vi "LAS.vi"() -> ()   [LabVIEW 2014, in "Panels.lvlib"]
uses:
  Panels.lvlib
  CSlibraries-extern/DimLVEvent/DimIndicators/DimIndicators.lvlib
  CSCore/CSSystem/CoreLib/CoreLib.lvlib
  CSlibraries/UtilityLib/UtilityLib.valueStatus.ctl
  CSlibraries/UtilityLib/UtilityLib.lvlib
  CSlibraries-extern/DimLVEvent/LVDimInterface/LVDimInterface.lvlib
  Instance           1 11Saved   LAS .vi
  CSlibraries-extern/DimLVEvent/DimIndicators/DimIndicators.numericType.ctl
  CSlibraries-extern/DimLVEvent/DimIndicators/DimIndicators.numericArrayType.ctl
  CSlibraries-extern/DimLVEvent/DimIndicators/DimIndicators.anyType.ctl
panel:
  in  "LASOuterQ-_SetValueInfoData":T1={"data"=[], "no link"=TRUE, "quality"=-1, "timeStamp"=0.0}
  in  "LASOuterQ+_SetValueInfoData":T1={"data"=[], "no link"=TRUE, "quality"=-1, "timeStamp"=0.0}
  in  "LASInnerQ-_SetValueInfoData":T1={"data"=[], "no link"=TRUE, "quality"=-1, "timeStamp"=0.0}
  in  "LASOuterQ-_SetData":T1={"data"=[], "no link"=TRUE, "quality"=-1, "timeStamp"=0.0}
  in  "LASOuterQ+_SetData":T1={"data"=[], "no link"=TRUE, "quality"=-1, "timeStamp"=0.0}
  in  "LASInnerQ-_SetData":T1={"data"=[], "no link"=TRUE, "quality"=-1, "timeStamp"=0.0}
  in  "LASOuterQ-_MonData":T2={"data"=inf, "no link"=TRUE, "quality"=-1, "timeStamp"=0.0}
  in  "LASOuterQ+_MonData":T2={"data"=inf, "no link"=TRUE, "quality"=-1, "timeStamp"=0.0}
  in  "LASInnerQ-_MonData":T2={"data"=inf, "no link"=TRUE, "quality"=-1, "timeStamp"=0.0}
  in  "LASOuterQ-":bool
  in  "LASOuterQ+":bool
  out "LASOuterQ+_Mon":dbl=inf format="%.4f"
  out "LASOuterQ-_Mon":dbl=inf format="%.4f"
  in  "LASInnerQ+":bool
  in  "LASAccel2":bool
  out "LASAccel2_Mon":dbl=inf format="%.4f"
  in  "LASInnerQ-":bool
  out "LASInnerQ-_Mon":dbl=inf format="%.4f"
  in  "SetFileLocation_Data":T3={"data"="NOLINK", "no link"=TRUE, "quality"=-1, "timeStamp"=0.0}
  in  "SetFileLocation":path=path "\\\\intranet\\Files/projects/lebit/Data Exchange/data/PenningEjectControl"
  in  "LASAccel3":bool
  in  "LASAccel4":bool
  in  "LASAccel1":bool
  out "LASAccel4_Mon":dbl=inf format="%.4f"
  out "LASAccel3_Mon":dbl=inf format="%.4f"
  out "i ref out":refnum<vi>
  in  "Last Loaded File_Data":T3={"data"="NOLINK", "no link"=TRUE, "quality"=-1, "timeStamp"=0.0}
  out "FileUpToDate":bool=TRUE caption="Parameter Changed"
  in  "Close All Panels":bool
  in  "LASAccel2_SetValueInfoData":T1={"data"=[], "no link"=TRUE, "quality"=-1, "timeStamp"=0.0}
  in  "LASAccel3_SetValueInfoData":T1={"data"=[], "no link"=TRUE, "quality"=-1, "timeStamp"=0.0}
  in  "LASAccel4_SetValueInfoData":T1={"data"=[], "no link"=TRUE, "quality"=-1, "timeStamp"=0.0}
  in  "LASInnerQ+_SetValueInfoData":T1={"data"=[], "no link"=TRUE, "quality"=-1, "timeStamp"=0.0}
  in  "LASAccel1_SetValueInfoData":T1={"data"=[], "no link"=TRUE, "quality"=-1, "timeStamp"=0.0}
  in  "LASAccel1_SetData":T1={"data"=[], "no link"=TRUE, "quality"=-1, "timeStamp"=0.0}
  in  "LASInnerQ+_SetData":T1={"data"=[], "no link"=TRUE, "quality"=-1, "timeStamp"=0.0}
  in  "LASAccel4_SetData":T1={"data"=[], "no link"=TRUE, "quality"=-1, "timeStamp"=0.0}
  in  "LASAccel3_SetData":T1={"data"=[], "no link"=TRUE, "quality"=-1, "timeStamp"=0.0}
  in  "LASAccel2_SetData":T1={"data"=[], "no link"=TRUE, "quality"=-1, "timeStamp"=0.0}
  out "Last Loaded File":string
  in  "LASInnerQ+_MonData":T2={"data"=inf, "no link"=TRUE, "quality"=-1, "timeStamp"=0.0}
  in  "LASAccel4_MonData":T2={"data"=inf, "no link"=TRUE, "quality"=-1, "timeStamp"=0.0}
  in  "LASAccel3_MonData":T2={"data"=inf, "no link"=TRUE, "quality"=-1, "timeStamp"=0.0}
  in  "LASAccel2_MonData":T2={"data"=inf, "no link"=TRUE, "quality"=-1, "timeStamp"=0.0}
  in  "LASAccel1_MonData":T2={"data"=inf, "no link"=TRUE, "quality"=-1, "timeStamp"=0.0}
  out "LASAccel1_Mon":dbl=inf format="%.4f"
  out "LASInnerQ+_Mon":dbl=inf format="%.4f"
  # "Parameter changed, data file is no longer up-to-date."
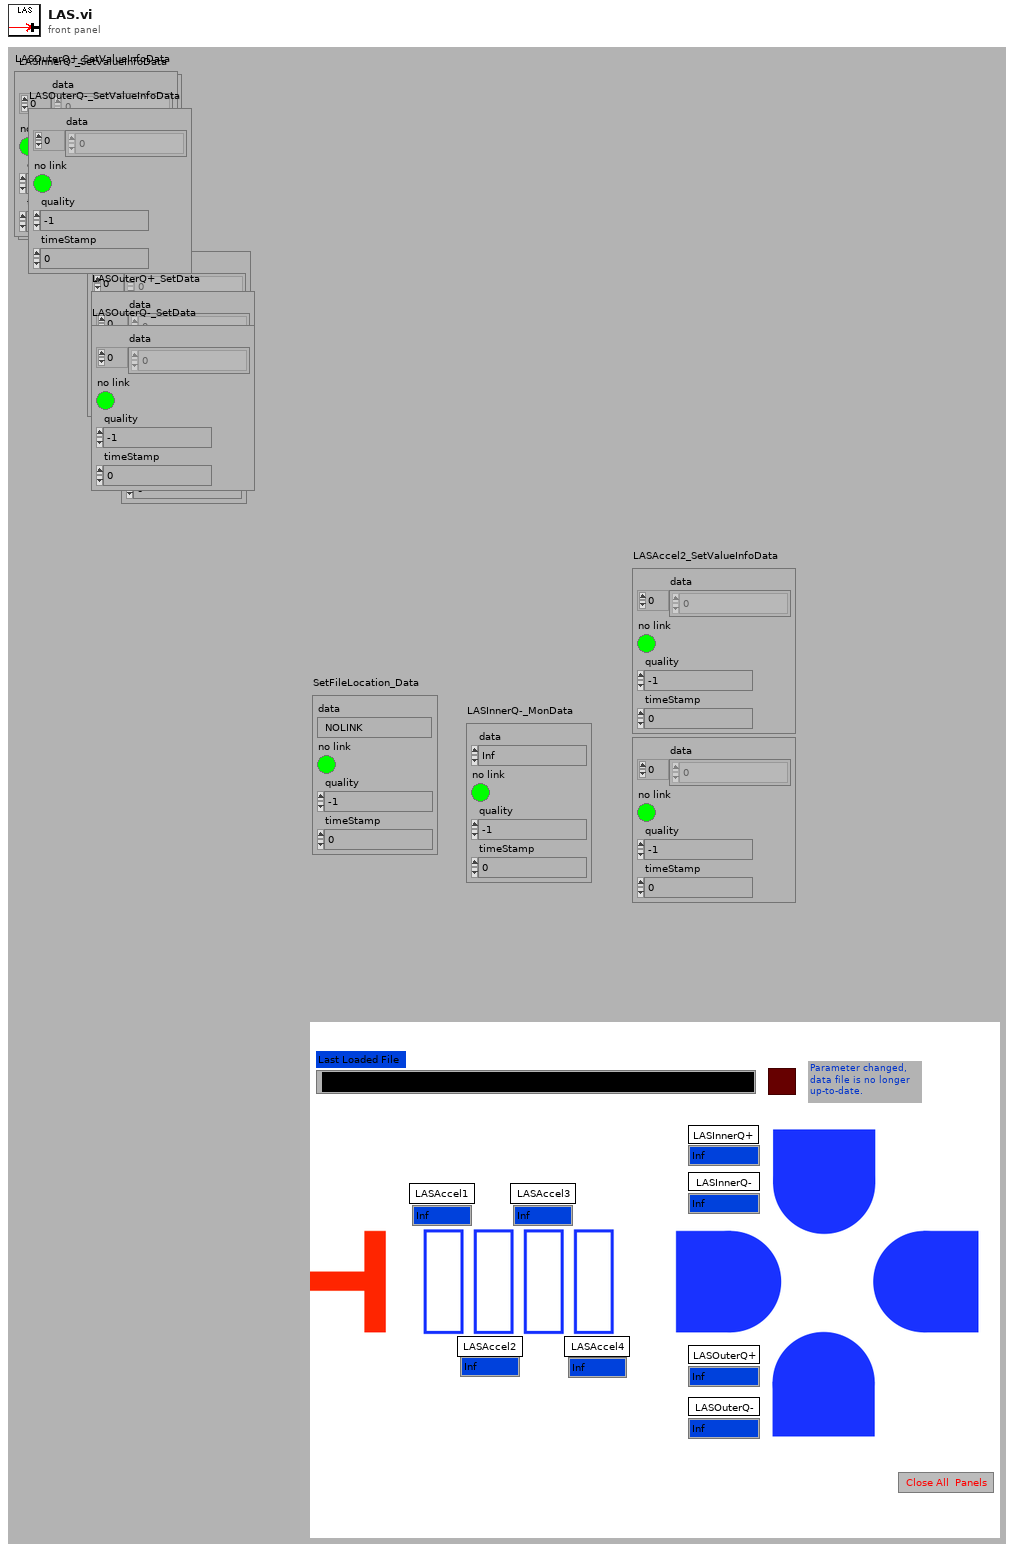
[diagram p1: front panel]
types:
  T1 = typedef "DimIndicators.lvlib/DimIndicators.numericArrayType.ctl" = cluster{"data":dbl[], "no link":bool, "quality":i32, "timeStamp":dbl}
  T2 = typedef "DimIndicators.lvlib/DimIndicators.numericType.ctl" = cluster{"data":dbl, "no link":bool, "quality":i32, "timeStamp":dbl}
  T3 = typedef "DimIndicators.lvlib/DimIndicators.anyType.ctl" = cluster{"data":string, "no link":bool, "quality":i32, "timeStamp":dbl}
  T4 = typedef "UtilityLib.lvlib/UtilityLib.valueStatus.ctl" = enum16{"no info available", "stand by/off", "on", "warning", "alarm/malfunction", "not implemented", "user action required", "important information", "system default", "control default", "indicator default", "button default"}
  T5 = cluster{"data":string, "no link":bool, "quality":i32, "timeStamp":dbl}
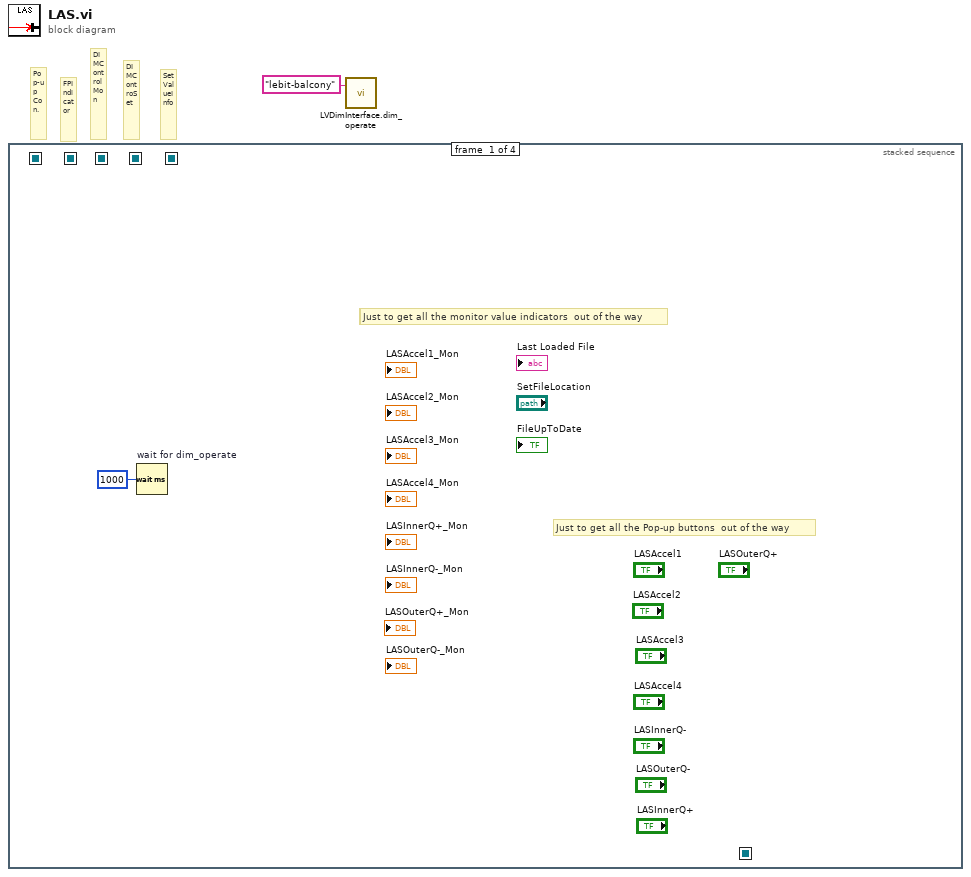
[diagram p0: block diagram]
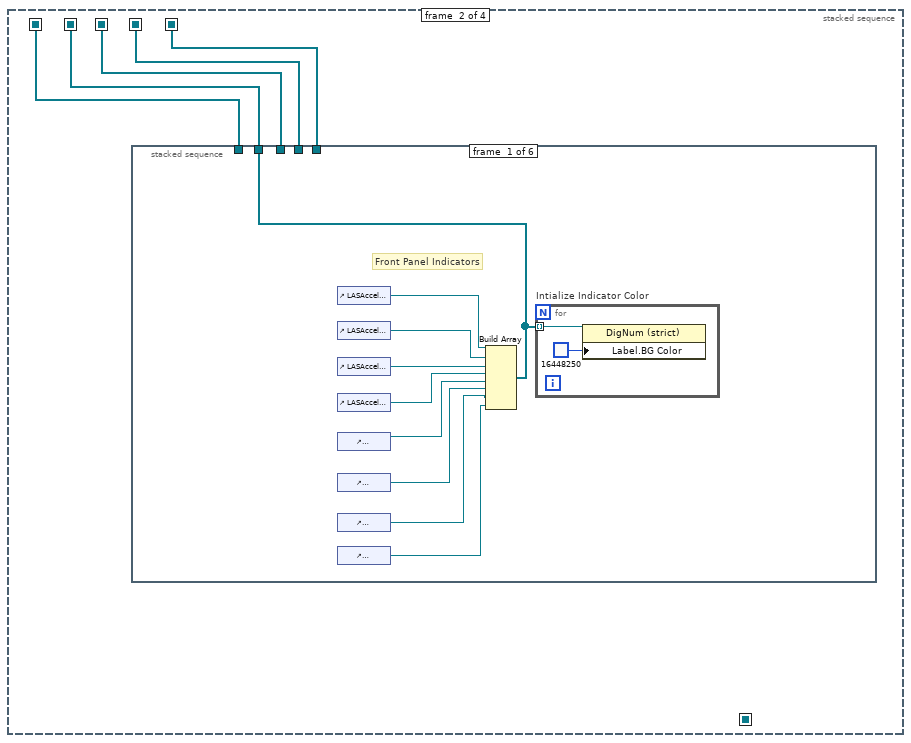
[diagram p2: hidden frame]
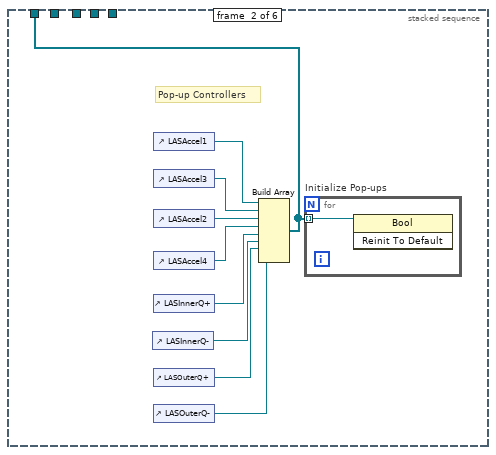
[diagram p3: hidden frame]
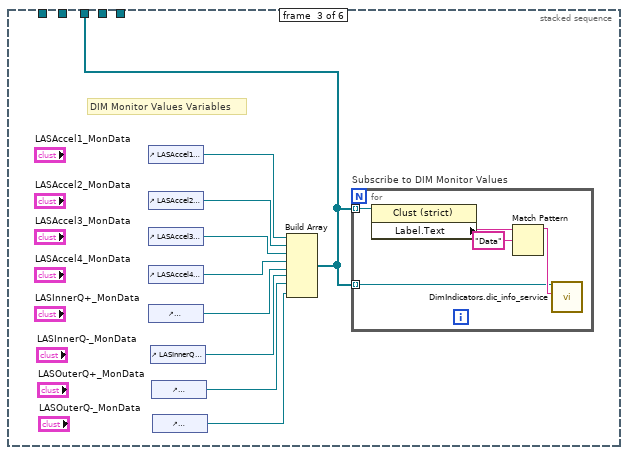
[diagram p4: hidden frame]
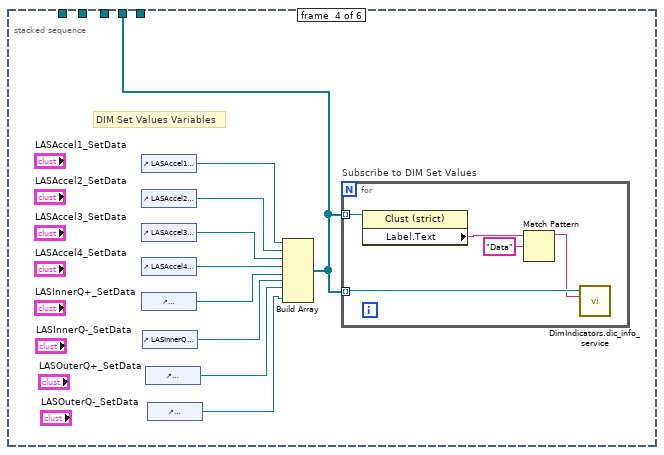
[diagram p5: hidden frame]
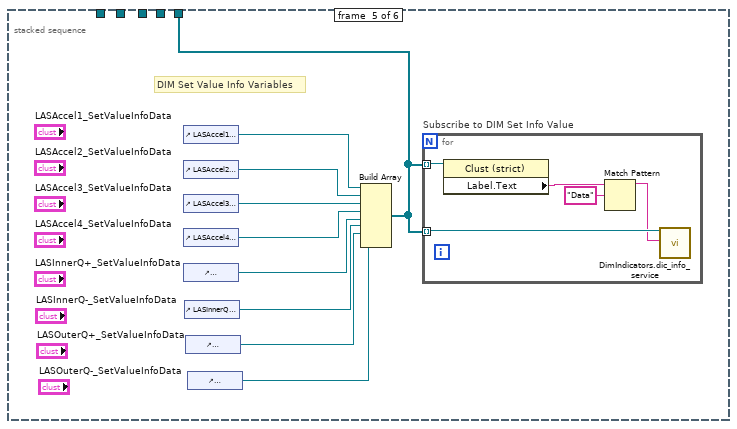
[diagram p6: hidden frame]
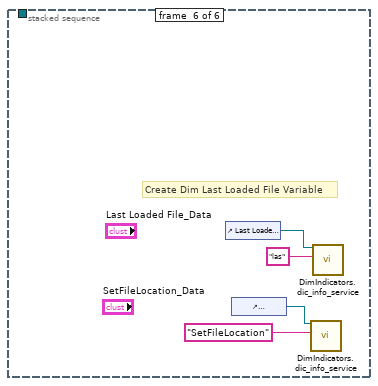
[diagram p7: hidden frame]
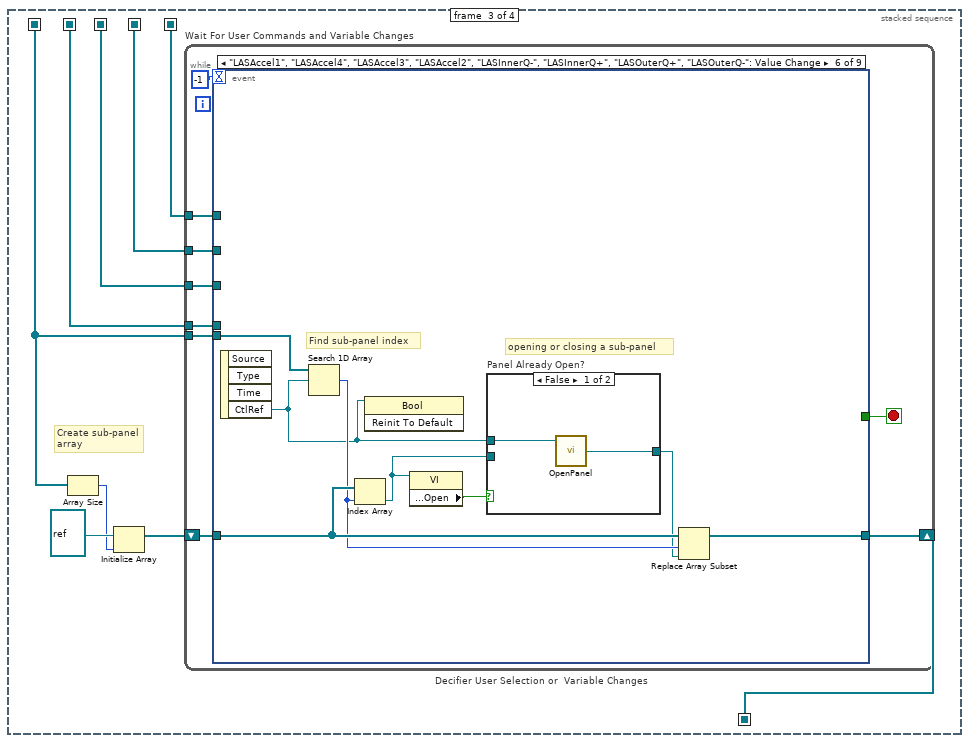
[diagram p8: hidden frame]
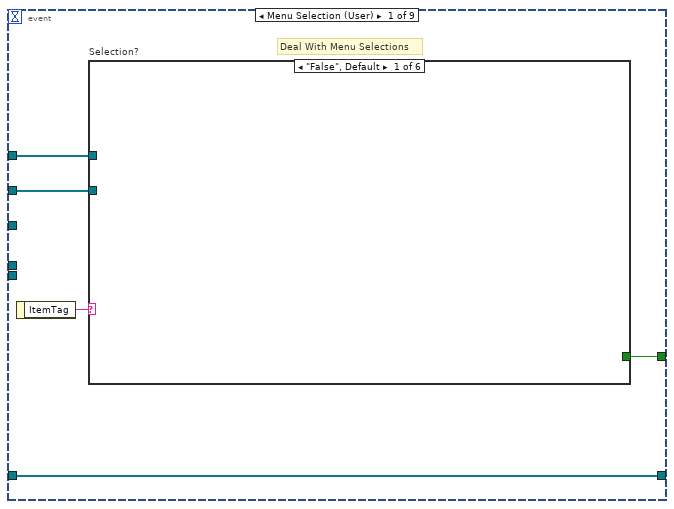
[diagram p9: hidden frame]
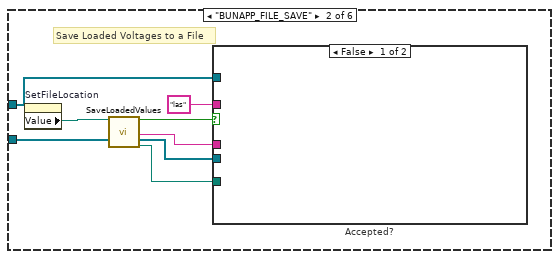
[diagram p10: hidden frame]
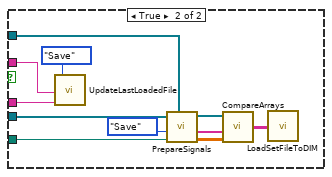
[diagram p11: hidden frame]
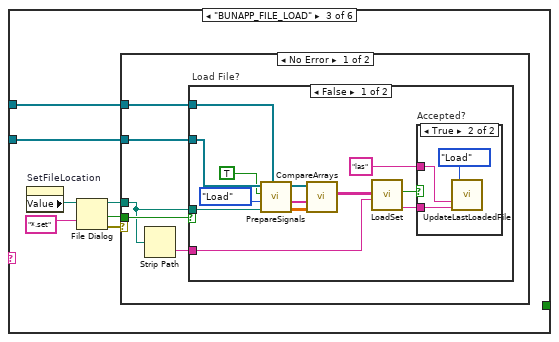
[diagram p12: hidden frame]
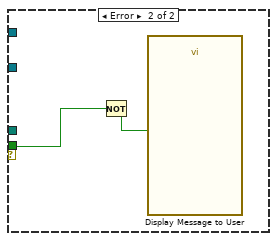
[diagram p15: hidden frame]
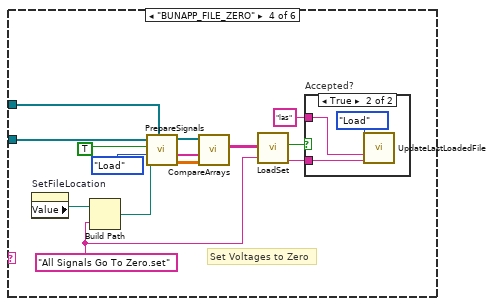
[diagram p16: hidden frame]
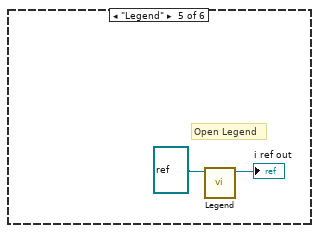
[diagram p18: hidden frame]
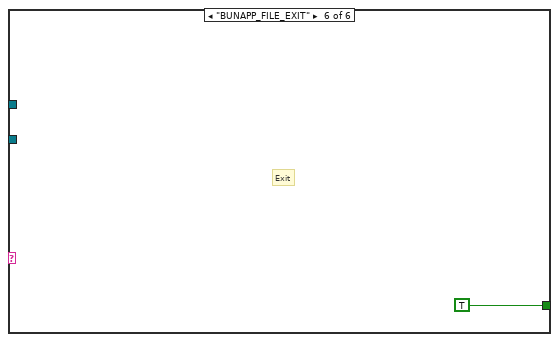
[diagram p19: hidden frame]
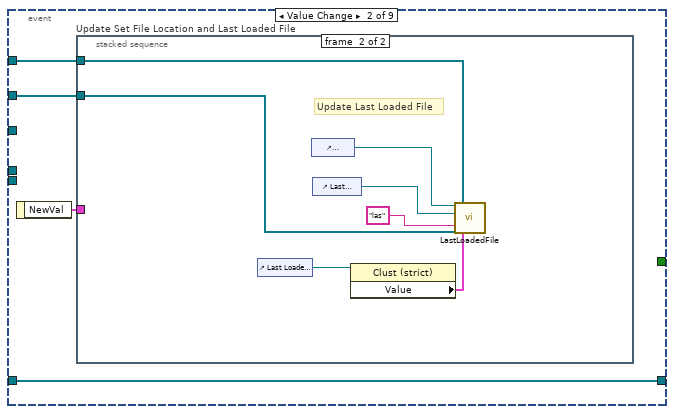
[diagram p20: hidden frame]
diagram:
  # "Pop-up Con."
  # "SetValueInfo"
  # "DIMControSet"
  # "DIMControlMon"
  # "FPIndicator"
  n1 = stacked-sequence {
    seq-local: [_ w7 _ _] -> [_ _ w80 _]
    seq-local: [_ w5 _ _] -> [_ _ w83 w279]
    seq-local: [_ _ w78 _] -> [_ _ _ w278]
    seq-local: [_ w4 _ _] -> [_ _ w77 w280]
    seq-local: [_ w3 _ _] -> [_ _ w76 w281]
    seq-local: [_ w6 _ _] -> [_ _ w75 _]
    frame #0 {
      # "Just to get all the monitor value indicators  out of the way"
      # "Just to get all the Pop-up buttons  out of the way"
      # "Just to get all the monitor value indicators  out of the way"
      n2 = Wait (ms) "wait for dim_operate"(milliseconds to wait=u32 1000) -> ()  [unwired: 1 out]
    }
    frame #1 {
      # "Arrange references to all monitor-value related buttons into an array."
      n3 = stacked-sequence {
        tunnel: [w14 _ _ _ _ _] -> w7
        tunnel: [_ w24 _ _ _ _] -> w6
        tunnel: [_ _ w32 _ _ _] -> w5
        tunnel: [_ _ _ w46 _ _] -> w4
        tunnel: [_ _ _ _ w60 _] -> w3
        frame #0 {
          # "Front Panel Indicators"
          n4 = control-ref of="LASAccel1_Mon"() -> (w13:refnum<vi>)
          n5 = control-ref of="LASAccel2_Mon"() -> (w10:refnum<vi>)
          n6 = control-ref of="LASAccel3_Mon"() -> (w12:refnum<vi>)
          n7 = control-ref of="LASAccel4_Mon"() -> (w15:refnum<vi>)
          n8 = control-ref of="LASInnerQ+_Mon"() -> (w16:refnum<vi>)
          n9 = control-ref of="LASInnerQ-_Mon"() -> (w11:refnum<vi>)
          n10 = control-ref of="LASOuterQ+_Mon"() -> (w9:refnum<vi>)
          n11 = control-ref of="LASOuterQ-_Mon"() -> (w8:refnum<vi>)
          n12 = Build Array(w13, w10, w12, w15, w16, w11, w9, w8) -> (w14:refnum<vi>[])
          n13 = for "Intialize Indicator Color" {
            tunnel: w14 -> [w18] mode=indexing
            n14 = property class="DigNum (strict)"(reference=w18, "Label.BG Color"=u32 16448250 ("Color Box")) -> ()  [unwired: 1 in, 2 out]
          }
        }
        frame #1 {
          # "Pop-up Controllers"
          n15 = control-ref of="LASInnerQ-"() -> (w20:refnum<vi>)
          n16 = control-ref of="LASAccel1"() -> (w27:refnum<vi>)
          n17 = control-ref of="LASAccel3"() -> (w26:refnum<vi>)
          n18 = control-ref of="LASAccel2"() -> (w23:refnum<vi>)
          n19 = control-ref of="LASAccel4"() -> (w25:refnum<vi>)
          n20 = control-ref of="LASInnerQ+"() -> (w22:refnum<vi>)
          n21 = control-ref of="LASOuterQ+"() -> (w21:refnum<vi>)
          n22 = control-ref of="LASOuterQ-"() -> (w19:refnum<vi>)
          n23 = Build Array(w27, w26, w23, w25, w22, w20, w21, w19) -> (w24:refnum<vi>[])
          n24 = for "Initialize Pop-ups" {
            tunnel: w24 -> [w28] mode=indexing
            n25 = invoke class="Bool" method="Reinit To Default"(reference=w28) -> ()  [unwired: 2 in, 3 out]
          }
        }
        frame #2 {
          # "DIM Monitor Values Variables"
          n26 = control-ref of="LASAccel1_MonData"() -> (w37:refnum<vi>)
          n27 = control-ref of="LASAccel2_MonData"() -> (w36:refnum<vi>)
          n28 = control-ref of="LASAccel3_MonData"() -> (w35:refnum<vi>)
          n29 = control-ref of="LASAccel4_MonData"() -> (w34:refnum<vi>)
          n30 = control-ref of="LASInnerQ+_MonData"() -> (w33:refnum<vi>)
          n31 = control-ref of="LASInnerQ-_MonData"() -> (w31:refnum<vi>)
          n32 = control-ref of="LASOuterQ+_MonData"() -> (w30:refnum<vi>)
          n33 = control-ref of="LASOuterQ-_MonData"() -> (w29:refnum<vi>)
          n34 = Build Array(w37, w36, w35, w34, w33, w31, w30, w29) -> (w32:refnum<vi>[])
          n35 = for "Subscribe to DIM Monitor Values" {
            tunnel: w32 -> [w39] mode=indexing
            tunnel: w32 -> [w38] mode=indexing
            n36 = property class="Clust (strict)"(reference=w38) -> ("Label.Text"=w41:string)  [unwired: 1 in, 2 out]
            n37 = Match Pattern(string=w41, regular expression="Data") -> (before substring=w40:string)  [unwired: 1 in, 3 out]
            n38 = call "DimIndicators.dic_info_service.vi"("controlRef"=w39, "serviceName"=w40) -> ()  [unwired: 16 in, 2 out]
          }
        }
        frame #3 {
          # "DIM Set Values Variables"
          n39 = control-ref of="LASAccel1_SetData"() -> (w51:refnum<vi>)
          n40 = control-ref of="LASAccel2_SetData"() -> (w50:refnum<vi>)
          n41 = control-ref of="LASAccel3_SetData"() -> (w49:refnum<vi>)
          n42 = control-ref of="LASAccel4_SetData"() -> (w48:refnum<vi>)
          n43 = control-ref of="LASInnerQ+_SetData"() -> (w47:refnum<vi>)
          n44 = control-ref of="LASInnerQ-_SetData"() -> (w45:refnum<vi>)
          n45 = control-ref of="LASOuterQ+_SetData"() -> (w44:refnum<vi>)
          n46 = control-ref of="LASOuterQ-_SetData"() -> (w43:refnum<vi>)
          n47 = Build Array(w51, w50, w49, w48, w47, w45, w44, w43) -> (w46:refnum<vi>[])
          n48 = for "Subscribe to DIM Set Values" {
            tunnel: w46 -> [w52] mode=indexing
            tunnel: w46 -> [w56] mode=indexing
            n49 = property class="Clust (strict)"(reference=w52) -> ("Label.Text"=w55:string)  [unwired: 1 in, 2 out]
            n50 = Match Pattern(string=w55, regular expression="Data") -> (before substring=w53:string)  [unwired: 1 in, 3 out]
            n51 = call "DimIndicators.dic_info_service.vi"("controlRef"=w56, "serviceName"=w53) -> ()  [unwired: 16 in, 2 out]
          }
        }
        frame #4 {
          # "DIM Set Value Info Variables"
          n52 = control-ref of="LASAccel1_SetValueInfoData"() -> (w65:refnum<vi>)
          n53 = control-ref of="LASAccel2_SetValueInfoData"() -> (w64:refnum<vi>)
          n54 = control-ref of="LASAccel3_SetValueInfoData"() -> (w63:refnum<vi>)
          n55 = control-ref of="LASAccel4_SetValueInfoData"() -> (w62:refnum<vi>)
          n56 = control-ref of="LASInnerQ+_SetValueInfoData"() -> (w61:refnum<vi>)
          n57 = control-ref of="LASInnerQ-_SetValueInfoData"() -> (w59:refnum<vi>)
          n58 = control-ref of="LASOuterQ+_SetValueInfoData"() -> (w58:refnum<vi>)
          n59 = control-ref of="LASOuterQ-_SetValueInfoData"() -> (w57:refnum<vi>)
          n60 = Build Array(w65, w64, w63, w62, w61, w59, w58, w57) -> (w60:refnum<vi>[])
          n61 = for "Subscribe to DIM Set Info Value" {
            tunnel: w60 -> [w66] mode=indexing
            tunnel: w60 -> [w70] mode=indexing
            n62 = property class="Clust (strict)"(reference=w66) -> ("Label.Text"=w69:string)  [unwired: 1 in, 2 out]
            n63 = Match Pattern(string=w69, regular expression="Data") -> (before substring=w67:string)  [unwired: 1 in, 3 out]
            n64 = call "DimIndicators.dic_info_service.vi"("controlRef"=w70, "serviceName"=w67) -> ()  [unwired: 16 in, 2 out]
          }
        }
        frame #5 {
          # "Create Dim Last Loaded File Variable"
          n65 = control-ref of="Last Loaded File_Data"() -> (w73:refnum<vi>)
          n66 = control-ref of="SetFileLocation_Data"() -> (w71:refnum<vi>)
          n67 = call "DimIndicators.dic_info_service.vi"("controlRef"=w71, "serviceName"="SetFileLocation" ("string")) -> ()  [unwired: 16 in, 2 out]
          n68 = call "DimIndicators.dic_info_service.vi"("controlRef"=w73, "serviceName"="las" ("string")) -> ()  [unwired: 16 in, 2 out]
        }
      }
    }
    frame #2 {
      # "Create sub-panel\narray"
      n69 = Array Size(array=w75) -> (size(s)=w79:i32)
      n70 = Initialize Array(refnum<vi> refnum ("vi reference"), w79) -> (w82:refnum<vi>[])
      n71 = while "Wait For User Commands and Variable Changes" {
        tunnel: w83 -> [w91]
        tunnel: w80 -> [w90]
        shift-right: [w88] -> w78
        shift-left: w82 -> [w89]
        tunnel: w77 -> [w87]
        tunnel: w76 -> [w86]
        tunnel: w75 -> [w84]
        stop <- w92 stop-if-true
        n72 = event "Decifier User Selection or  Variable Changes" shown="[5] \"LASAccel1\", \"LASAccel4\", \"LASAccel3\", \"LASAccel2\", \"LASInnerQ-\", \"LASInnerQ+\", \"LASOuterQ+\", \"LASOuterQ-\": Value Change" {
          selector: _ -> [_ _ _ _ _ _ _ _ _]
          dyn-events: _ -> [_ _ _ _ _ _ _ _ _]
          timeout: -1 -> [_ _ _ _ _ _ _ _ _]
          tunnel: [w94 _ _ _ _ _ _ _ TRUE ("stop")] -> w92
          tunnel: w91 -> [_ _ _ _ _ _ _ _ w254]
          tunnel: w90 -> [_ _ _ w204 _ _ _ _ _]
          tunnel: w89 -> [w97 w169 w201 w203 w231 w239 w246 w252 w253]
          tunnel: [w97 w169 w201 w203 w231 w237 w244 w252 _] -> w88
          tunnel: w87 -> [w95 w168 w198 _ w228 _ _ _ w255]
          tunnel: w86 -> [w93 w167 w195 _ _ _ _ _ w256]
          tunnel: w84 -> [_ _ _ _ _ w233 _ _ _]
          event Menu Selection (User) {
            # "Deal With Menu Selections"
            n73 = event-data() -> ("ItemTag"=w96:string)  [unwired: 1 in]
            n74 = case "Selection?" shown="\"False\", Default" w96 {
              tunnel: w95 -> [_ w102 w122 w160 _ _]
              tunnel: [_ _ _ _ _ TRUE ("stop")] -> w94
              tunnel: w93 -> [_ w98 w117 w147 _ _]
              frame "False", Default {
              }
              frame "BUNAPP_FILE_SAVE" {
                # "Save Loaded Voltages to a File"
                n75 = property on="SetFileLocation" class="Path"() -> ("Value"=w103:path)  [unwired: 2 in, 2 out]
                n76 = call "SaveLoadedValues.vi"("Panel Location?"=w103, "DIMControlSet in"=w102) -> ("File Saved?"=w104:bool, "File Name"=w101:string, "DIMControlSet out"=w99:refnum<vi>[], "Path"=w100:path)  [unwired: 14 in]
                n77 = case "Accepted?" shown="False" w104 {
                  tunnel: w101 -> [_ w114]
                  tunnel: "las" ("string") -> [_ w116]
                  tunnel: w99 -> [_ w115]
                  tunnel: w100 -> [_ w113]
                  tunnel: w98 -> [_ w107]
                  frame False {
                  }
                  frame True {
                    n78 = call "UpdateLastLoadedFile.vi"("LoadOrSave"=enum16{"Load", "Save"}."Save", "GUIName"=w116, "FileNameIn"=w114) -> ()  [unwired: 13 in]
                    n79 = call "PrepareSignals.vi"("SetValueInfo in"=w107, "setfile path"=w113, "Enum"=enum16{"Save", "Load"}."Save", "DIMControSet in"=w115) -> ("indexed loaded Array"=w111:dbl[][], "Name Array"=w112:string[], "DIMControSet out"=w110:refnum<vi>[])  [unwired: 5 in]
                    n80 = call "CompareArrays.vi"("indexed loaded Array"=w111, "Name Array"=w112, "DIMControSet"=w110) -> ("Table for loading values"=w109:string[][])  [unwired: 4 in]
                    n81 = call "LoadSetFileToDIM.vi"("output array"=w109) -> ()  [unwired: 2 in]
                  }
                }
              }
              frame "BUNAPP_FILE_LOAD" {
                # "Promt User For File to Load"
                n82 = property on="SetFileLocation" class="Path"() -> ("Value"=w119:path)  [unwired: 2 in, 2 out]
                n83 = File Dialog(6:"*.set" ("pattern (all files)"), 11:w119) -> (0:w118:errorcluster, 1:w123:bool, 3:w120:path)  [unwired: 5 in, 1 out]
                n84 = case shown="No Error" w118 {
                  tunnel: w123 -> [w128 w145]
                  tunnel: w122 -> [w127 _]
                  tunnel: w120 -> [w125 _]
                  tunnel: w117 -> [w124 _]
                  frame No Error {
                    n85 = Strip Path(path=w125) -> (name=w126:string)  [unwired: 1 out]
                    n86 = case "Load File?" shown="False" w128 {
                      tunnel: w127 -> [w141 _]
                      tunnel: w126 -> [w135 _]
                      tunnel: w125 -> [w136 _]
                      tunnel: w124 -> [w129 _]
                      frame False {
                        n87 = call "PrepareSignals.vi"("SetValueInfo in"=w129, "setfile path"=w136, "Enum"=enum16{"Save", "Load"}."Load", "Display Message to \nUser"=TRUE ("Display Message to \nUser"), "DIMControSet in"=w141) -> ("indexed loaded Array"=w139:dbl[][], "Name Array"=w138:string[], "DIMControSet out"=w140:refnum<vi>[])  [unwired: 4 in]
                        n88 = call "CompareArrays.vi"("indexed loaded Array"=w139, "Name Array"=w138, "DIMControSet"=w140) -> ("Table for loading values"=w137:string[][])  [unwired: 4 in]
                        n89 = call "LoadSet.vi"("File Name In"=w135, "output array"=w137) -> ("File Name out"=w134:string, "Accepted"=w133:bool)  [unwired: 8 in]
                        n90 = case "Accepted?" shown="True" w133 {
                          tunnel: w134 -> [_ w144]
                          tunnel: "las" ("string") -> [_ w143]
                          frame False {
                          }
                          frame True {
                            n91 = call "UpdateLastLoadedFile.vi"("LoadOrSave"=enum16{"Load", "Save"}."Load", "GUIName"=w143, "FileNameIn"=w144) -> ()  [unwired: 13 in]
                          }
                        }
                      }
                      frame True {
                      }
                    }
                  }
                  frame Error {
                    n92 = Not(x=w145) -> (.not. x?=w146:bool)
                    n93 = call "Display Message to User"("Enable"=w146) -> ()  [unwired: 9 in, 2 out]
                  }
                }
              }
              frame "BUNAPP_FILE_ZERO" {
                w151 = "All Signals Go To Zero.set" ("File Name")
                # "Set Voltages to Zero"
                n94 = property on="SetFileLocation" class="Path"() -> ("Value"=w149:path)  [unwired: 2 in, 2 out]
                n95 = Build Path(base path=w149, name or relative path=w151) -> (appended path=w150:path)
                n96 = call "PrepareSignals.vi"("SetValueInfo in"=w147, "setfile path"=w150, "Enum"=enum16{"Save", "Load"}."Load", "Display Message to \nUser"=TRUE ("Display Message to \nUser"), "DIMControSet in"=w160) -> ("indexed loaded Array"=w158:dbl[][], "Name Array"=w157:string[], "DIMControSet out"=w159:refnum<vi>[])  [unwired: 4 in]
                n97 = call "CompareArrays.vi"("indexed loaded Array"=w158, "Name Array"=w157, "DIMControSet"=w159) -> ("Table for loading values"=w156:string[][])  [unwired: 4 in]
                n98 = call "LoadSet.vi"("File Name In"=w151, "output array"=w156) -> ("File Name out"=w154:string, "Accepted"=w155:bool)  [unwired: 8 in]
                n99 = case "Accepted?" shown="True" w155 {
                  tunnel: w154 -> [_ w163]
                  tunnel: "las" ("string") -> [_ w162]
                  frame False {
                  }
                  frame True {
                    n100 = call "UpdateLastLoadedFile.vi"("LoadOrSave"=enum16{"Load", "Save"}."Load", "GUIName"=w162, "FileNameIn"=w163) -> ()  [unwired: 13 in]
                  }
                }
              }
              frame "Legend" {
                # "Open Legend"
                n101 = call "Legend.vi"("i ref in"=refnum<vi> refnum) -> ("i ref out"=→"i ref out":refnum<vi>)  [unwired: 10 in]
              }
              frame "BUNAPP_FILE_EXIT" {
                # "Exit"
              }
            }
          }
          event Value Change {
            n102 = event-data() -> ("NewVal"=w170:T3)  [unwired: 1 in]
            n103 = stacked-sequence "Update Set File Location and Last Loaded File" {
              tunnel: w170 -> [w172 _]
              tunnel: w168 -> [_ w192]
              tunnel: w167 -> [_ w188]
              frame #0 {
                # "Update Set File Location"
                n104 = Unbundle By Name(w172) -> ("data"=w181:string, "no link"=w180:bool, "quality"=w179:i32)
                n105 = case "Link?" shown="False" w180 {
                  tunnel: w179 -> [w185 _]
                  tunnel: [w184 UtilityLib.valueStatus."no info available" ("valueStatus")] -> w182
                  tunnel: w181 -> [w183 _]
                  tunnel: [w183 w186] -> w177
                  frame False {
                    n106 = call "CoreLib.quality 2 status.vi"("quality"=w185) -> ("valueStatus"=w184:T4)  [unwired: 18 in]
                  }
                  frame True {
                    n107 = call "EmptyString.vi"() -> ("String"=w186:string)
                  }
                }
                n108 = Type Cast(type="" ("regular expression"), x=w177) -> (*(type *) &x=w176:string)
                n109 = String To Path(string=w176) -> (path=w173:path)
                n110 = control-ref of="SetFileLocation"() -> (w171:refnum<vi>)
                n111 = Build Path(base path=w173, name or relative path="LASControl") -> (appended path=w174:path)
                n112 = property class="Path"(reference=w171, "Value"=w174) -> ()  [unwired: 1 in, 2 out]
                n113 = call "UtilityLib.set color of GUI object.vi"("GUI object Ref"=w171, "valueStatus"=w182) -> ()  [unwired: 17 in, 1 out]
              }
              frame #1 {
                # "Update Last Loaded File"
                n114 = control-ref of="Last Loaded File_Data"() -> (w189:refnum<vi>)
                n115 = control-ref of="SetFileLocation"() -> (w191:refnum<vi>)
                n116 = control-ref of="Last Loaded File"() -> (w190:refnum<vi>)
                n117 = property class="Clust (strict)"(reference=w189) -> ("Value"=w194:T5)  [unwired: 1 in, 2 out]
                n118 = call "LastLoadedFile.vi"("SetFileLocation"=w191, "Last Loaded File"=w190, "GUIName"="las" ("string"), "DIMControSet in"=w192, "SetValueInfo in"=w188, "NewVal"=w194) -> ()  [unwired: 14 in]
              }
            }
          }
          event Value Change {
            # "Update Last Loaded File"
            n119 = event-data() -> ("NewVal"=w200:T3)  [unwired: 1 in]
            n120 = control-ref of="SetFileLocation"() -> (w197:refnum<vi>)
            n121 = control-ref of="Last Loaded File"() -> (w196:refnum<vi>)
            n122 = call "LastLoadedFile.vi"("SetFileLocation"=w197, "Last Loaded File"=w196, "GUIName"="las" ("string"), "DIMControSet in"=w198, "SetValueInfo in"=w195, "NewVal"=w200) -> ()  [unwired: 14 in]
          }
          event Value Change {
            n123 = event-data() -> ("CtlRef"=w202:refnum<vi>, "NewVal"=w205:T2)  [unwired: 1 in, 4 out]
            n124 = for "Check if Indicator Exists for the Monitor Value?" {
              tunnel: w205 -> [w214]
              tunnel: w204 -> [w211] mode=indexing
              tunnel: w202 -> [w210]
              # "Updating a Monitor Value"
              n125 = property class="DigNum (strict)"(reference=w211) -> (reference out=w206:refnum<vi>, "Label.Text"=w208:string)  [unwired: 1 in, 1 out]
              n126 = property class="Clust (strict)"(reference=w210) -> ("Label.Text"=w212:string)  [unwired: 1 in, 2 out]
              n127 = Match Pattern(string=w212, regular expression="Data") -> (before substring=w207:string)  [unwired: 1 in, 3 out]
              n128 = Equal?(x=w208, y=w207) -> (x = y?=w209:bool)
              n129 = case "Indicator exists?" shown="True" w209 {
                tunnel: w214 -> [w221 _]
                tunnel: w206 -> [w215 _]
                frame True {
                  n130 = Unbundle By Name(w221) -> ("data"=w217:dbl, "no link"=w218:bool, "quality"=w220:i32)
                  n131 = case shown="True" w218 {
                    tunnel: w220 -> [w224 _]
                    tunnel: [w223 UtilityLib.valueStatus."no info available" ("valueStatus")] -> w219
                    tunnel: w217 -> [w222 _]
                    tunnel: [w222 inf] -> w216
                    frame False {
                      n132 = call "CoreLib.quality 2 status.vi"("quality"=w224) -> ("valueStatus"=w223:T4)  [unwired: 18 in]
                    }
                    frame True {
                    }
                  }
                  n133 = property class="DigNum (strict)"(reference=w215, "Value"=w216) -> ()  [unwired: 1 in, 2 out]
                  n134 = call "TextColor.vi"("valueStatus"=w219, "reference"=w215) -> ()  [unwired: 10 in]
                }
                frame False {
                }
              }
            }
          }
          event Value Change {
            n135 = event-data() -> ("CtlRef"=w229:refnum<vi>)  [unwired: 1 in, 5 out]
            n136 = property on="FileUpToDate" class="Bool (strict)"() -> ("Value"=w227:bool)  [unwired: 2 in, 2 out]
            n137 = call "FileUpToDate.vi"("FileUpToDate in"=w227, "DIMControSet out"=w228, "CtlRef"=w229) -> ("FileUpToDate out"=w230:bool)  [unwired: 16 in]
            n138 = property on="FileUpToDate" class="Bool (strict)"("Value"=w230) -> ()  [unwired: 2 in, 2 out]
          }
          event "LASAccel1", "LASAccel4", "LASAccel3", "LASAccel2", "LASInnerQ-", "LASInnerQ+", "LASOuterQ+", "LASOuterQ-": Value Change {
            # "Find sub-panel index"
            # "opening or closing a sub-panel"
            n139 = event-data() -> ("CtlRef"=w232:refnum<vi>)  [unwired: 1 in, 3 out]
            n140 = Search 1D Array(1D array=w233, element=w232) -> (index of element=w238:i32)  [unwired: 1 in]
            n141 = Index Array(array=w239, index=w238) -> (element=w236:refnum<vi>)
            n142 = invoke class="Bool" method="Reinit To Default"(reference=w232) -> ()  [unwired: 2 in, 3 out]
            n143 = property class="VI"(reference=w236) -> ("Front Panel.Open"=w235:bool)  [unwired: 1 in, 2 out]
            n144 = case "Panel Already Open?" shown="False" w235 {
              tunnel: w232 -> [w240 _]
              tunnel: w236 -> [_ w243]
              tunnel: [w241 refnum<vi> refnum ("vi reference")] -> w234
              frame False {
                n145 = call "OpenPanel.vi"("CtlRef"=w240) -> ("vi reference"=w241:refnum<vi>)  [unwired: 2 in]
              }
              frame True {
                n146 = call "PanelClose.vi"("vi reference"=w243) -> ()
              }
            }
            n147 = Replace Array Subset(array=w239, new element=w234, index=w238) -> (w237:refnum<vi>[])
          }
          event "Close All Panels": Value Change {
            n148 = event-data() -> ()  [unwired: 1 in, 6 out]
            n149 = case "Close Open Panels?" shown="True" "Close All Panels" {
              tunnel: w246 -> [w247 w249]
              tunnel: [w247 w248] -> w244
              frame False {
              }
              frame True {
                n150 = for "Close Open Panels" {
                  tunnel: w249 -> [w251] mode=indexing
                  tunnel: w249 -> [w250]
                  tunnel: [w250] -> w248
                  n151 = call "PanelClose.vi"("vi reference"=w251) -> ()
                }
              }
            }
          }
          event Timeout {
            # "Timeout"
            n152 = event-data() -> ()  [unwired: 1 in, 3 out]
          }
          event Panel Close? {
            n153 = event-data() -> ()  [unwired: 1 in, 4 out]
            n154 = stacked-sequence {
              tunnel: w256 -> [w262 _]
              tunnel: w255 -> [w261 _]
              tunnel: w254 -> [w260 _]
              tunnel: w253 -> [w263 _]
              frame #0 {
                # "Release DIM Services"
                n155 = for "Close Open Panels" {
                  tunnel: w263 -> [w273] mode=indexing
                  n156 = call "PanelClose.vi"("vi reference"=w273) -> ()
                }
                n157 = for "For Each Service" {
                  tunnel: w262 -> [w271] mode=indexing
                  n158 = Not A Number/Path/Refnum?(number/path/refnum=w271) -> (NaN/Path/Refnum?=w270:bool)
                  n159 = case "Not a Reference?" shown="False" w270 {
                    tunnel: w271 -> [w272 _]
                    frame False {
                      n160 = call "DimIndicators.dic_release_service.vi"("controlRef"=w272) -> ()  [unwired: 18 in, 1 out]
                    }
                    frame True {
                    }
                  }
                }
                n161 = for "For Each Service" {
                  tunnel: w261 -> [w268] mode=indexing
                  n162 = Not A Number/Path/Refnum?(number/path/refnum=w268) -> (NaN/Path/Refnum?=w267:bool)
                  n163 = case "Not a Reference?" shown="False" w267 {
                    tunnel: w268 -> [w269 _]
                    frame False {
                      n164 = call "DimIndicators.dic_release_service.vi"("controlRef"=w269) -> ()  [unwired: 18 in, 1 out]
                    }
                    frame True {
                    }
                  }
                }
                n165 = for "For Each Service" {
                  tunnel: w260 -> [w265] mode=indexing
                  n166 = Not A Number/Path/Refnum?(number/path/refnum=w265) -> (NaN/Path/Refnum?=w264:bool)
                  n167 = case "Not a Reference?" shown="False" w264 {
                    tunnel: w265 -> [w266 _]
                    frame False {
                      n168 = call "DimIndicators.dic_release_service.vi"("controlRef"=w266) -> ()  [unwired: 18 in, 1 out]
                    }
                    frame True {
                    }
                  }
                }
                n169 = control-ref of="Last Loaded File_Data"() -> (w259:refnum<vi>)
                n170 = control-ref of="SetFileLocation_Data"() -> (w258:refnum<vi>)
                n171 = call "DimIndicators.dic_release_service.vi"("controlRef"=w259) -> ()  [unwired: 18 in, 1 out]
                n172 = call "DimIndicators.dic_release_service.vi"("controlRef"=w258) -> ()  [unwired: 18 in, 1 out]
              }
              frame #1 {
                # "Close Front Panel"
                n173 = Current VI's Path() -> (path=w274:path)
                n174 = Open VI Reference(vi path=w274) -> (vi reference=w276:refnum<vi>, error out=w277:errorcluster)  [unwired: 5 in]
                n175 = property class="VI"(reference=w276, error in=w277, "Front Panel Window:Open"=FALSE) -> ()  [unwired: 2 out]
              }
            }
            n176 = event-data() -> ()  [unwired: 2 in, 1 out]
          }
        }
      }
    }
    frame #3 {
      n177 = stacked-sequence {
        tunnel: w278 -> [w287 _ _]
        tunnel: w280 -> [w285 _ _]
        tunnel: w281 -> [w286 _ _]
        tunnel: w279 -> [w284 _ _]
        frame #0 {
          # "Release DIM Services"
          n178 = control-ref of="Last Loaded File_Data"() -> (w283:refnum<vi>)
          n179 = control-ref of="SetFileLocation_Data"() -> (w282:refnum<vi>)
          n180 = call "DimIndicators.dic_release_service.vi"("controlRef"=w283) -> ()  [unwired: 18 in, 1 out]
          n181 = call "DimIndicators.dic_release_service.vi"("controlRef"=w282) -> ()  [unwired: 18 in, 1 out]
          n182 = for "For Each Service" {
            tunnel: w286 -> [w295] mode=indexing
            n183 = Not A Number/Path/Refnum?(number/path/refnum=w295) -> (NaN/Path/Refnum?=w294:bool)
            n184 = case "Not a Reference?" shown="False" w294 {
              tunnel: w295 -> [w296 _]
              frame False {
                n185 = call "DimIndicators.dic_release_service.vi"("controlRef"=w296) -> ()  [unwired: 18 in, 1 out]
              }
              frame True {
              }
            }
          }
          n186 = for "For Each Service" {
            tunnel: w285 -> [w292] mode=indexing
            n187 = Not A Number/Path/Refnum?(number/path/refnum=w292) -> (NaN/Path/Refnum?=w291:bool)
            n188 = case "Not a Reference?" shown="False" w291 {
              tunnel: w292 -> [w293 _]
              frame False {
                n189 = call "DimIndicators.dic_release_service.vi"("controlRef"=w293) -> ()  [unwired: 18 in, 1 out]
              }
              frame True {
              }
            }
          }
          n190 = for "For Each Service" {
            tunnel: w284 -> [w289] mode=indexing
            n191 = Not A Number/Path/Refnum?(number/path/refnum=w289) -> (NaN/Path/Refnum?=w288:bool)
            n192 = case "Not a Reference?" shown="False" w288 {
              tunnel: w289 -> [w290 _]
              frame False {
                n193 = call "DimIndicators.dic_release_service.vi"("controlRef"=w290) -> ()  [unwired: 18 in, 1 out]
              }
              frame True {
              }
            }
          }
          n194 = for "Close Open Panels" {
            tunnel: w287 -> [w297] mode=indexing
            n195 = call "PanelClose.vi"("vi reference"=w297) -> ()
          }
        }
        frame #1 {
          # "Close Front Panel"
          n196 = Current VI's Path() -> (path=w301:path)
          n197 = Open VI Reference(vi path=w301) -> (vi reference=w299:refnum<vi>, error out=w298:errorcluster)  [unwired: 5 in]
          n198 = property class="VI"(reference=w299, error in=w298, "Front Panel Window:Open"=FALSE) -> ()  [unwired: 2 out]
        }
        frame #2 {
          # "Stop Panel"
          n199 = Stop(stop? (T)=TRUE) -> ()
        }
      }
    }
  }
  n200 = call "LVDimInterface.dim_operate.vi"("DNSNode"="lebit-balcony" ("DNS node")) -> ()  [unwired: 19 in]
